vi "get Property Value.vi"(7 "propertyName":string, 8 "error in":errorcluster, 9 "categoryName":string, 10 "resourceOrImageId":u32, 11 "cycloneHandle":u32) -> (0 "error out":errorcluster, 1 "categoryName out":string, 3 "function return":string, 5 "propertyName out":string)   [LabVIEW 2021, in "CycloneControlSDK.lvlib"]
doc: "extern \"C\" char * _cdecl getPropertyValue(uint32_t cycloneHandle, uint32_t resourceOrImageId, char *categoryName, char *propertyName);"
uses:
  CycloneControlSDK.lvlib
  CycloneControlSDK_64.dll
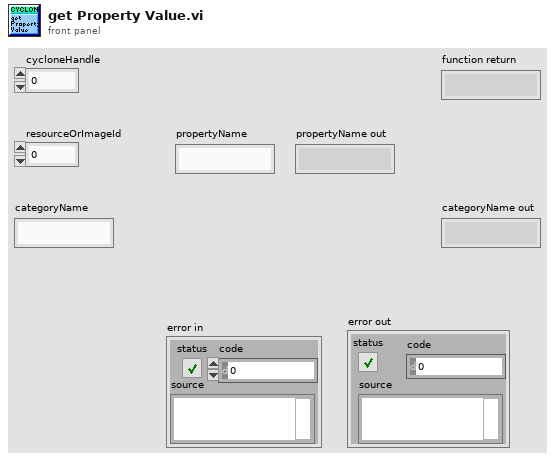
[diagram p1: front panel]
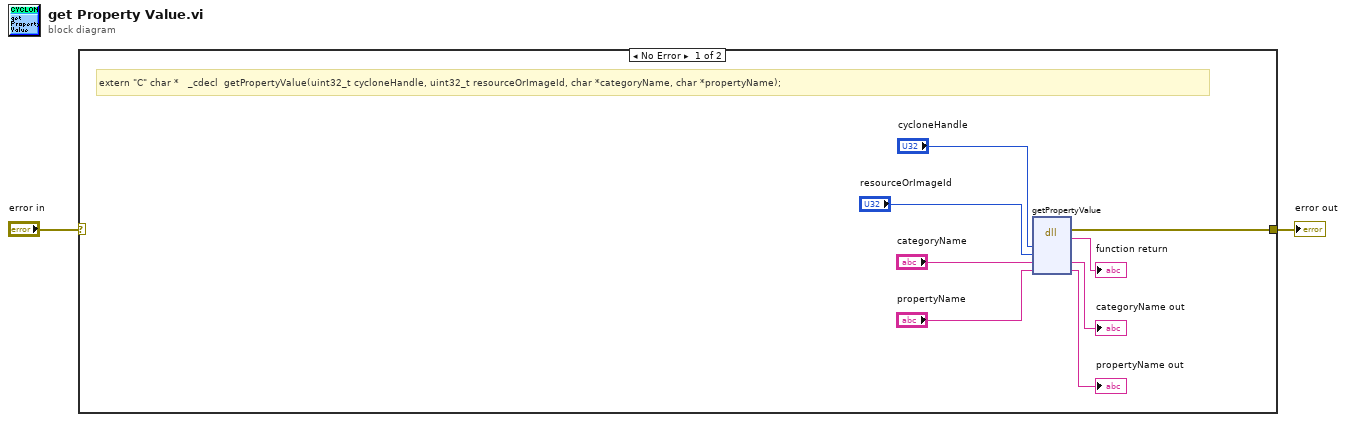
[diagram p0: block diagram]
diagram:
  n1 = case shown="No Error" "error in" {
    selector: "error in" -> [_ w11]
    tunnel: [w3 w11] -> w1
    frame No Error {
      # "extern \"C\" char *   _cdecl  getPropertyValue(uint32_t cycloneHandle, uint32_t resourceOrImageId, char *categoryName, char *propertyName);"
      n2 = dll-call lib="C:/PEMicro/cyclone/cycloneControl/controlsdk/examples/labview2018/user.lib/CycloneControlSDK/CycloneControlSDK_64.dll" fn="getPropertyValue"("cycloneHandle"="cycloneHandle", "resourceOrImageId"="resourceOrImageId", "categoryName"="categoryName", "propertyName"="propertyName") -> (error out=w3:errorcluster, "return type"=→"function return":string, "categoryName"=→"categoryName out":string, "propertyName"=→"propertyName out":string)  [unwired: 5 in, 1 out]
    }
    frame Error {
    }
  }
  "error out" <- w1
